vi "Error to String and Severity.vi"(8 "error in (no error)":errorcluster) -> (2 "Severity":T1, 3 "Error Text":string)   [LabVIEW 2016, in "LUL-SysLog.lvlib"]
uses:
  LUL-All/LUL-Syslog/CTL/SysLog Severity.ctl
  LUL-All/LUL-Syslog/LUL-SysLog.lvlib
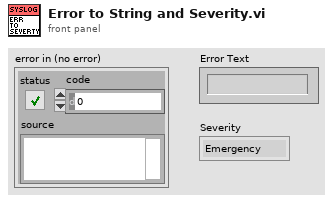
[diagram p1: front panel]
types:
  T1 = typedef "LUL-SysLog.lvlib/SysLog Severity.ctl" = enum16{"Emergency", "Alert", "Critical", "Error", "Wanring", "Notice", "Informational", "Debug"}
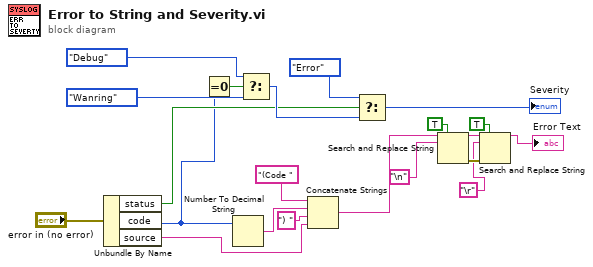
[diagram p0: block diagram]
diagram:
  n1 = Unbundle By Name("error in (no error)") -> ("status"=w15:bool, "code"=w2:i32, "source"=w18:string)
  n2 = Equal To 0?(x=w2) -> (x = 0?=w3:bool)
  n3 = Number To Decimal String(number=w2) -> (decimal integer string=w13:string)  [unwired: 1 in]
  n4 = Select(t=SysLog_Severity."Debug" ("Severity"), s=w3, f=SysLog_Severity."Wanring") -> (s? t:f=w21:T1)
  n5 = Concatenate Strings("(Code " ("string"), w13, ") " ("string"), w18) -> (w1:string)
  n6 = Select(t=SysLog_Severity."Error" ("Severity"), s=w15, f=w21) -> (s? t:f=→"Severity":T1)
  n7 = Search and Replace String(replace all?=TRUE ("replace all? (F)"), input string=w1, search string="\n") -> (result string=w7:string, error out=w8:errorcluster)  [unwired: 5 in, 2 out]
  n8 = Search and Replace String(replace all?=TRUE ("replace all? (F)"), input string=w7, search string="\r", error in=w8) -> (result string=→"Error Text":string)  [unwired: 4 in, 3 out]
